vi "Database Logging.vi"() -> ()   [LabVIEW 2011]
doc: "This example inserts data into a table named logging in the LabVIEW.mdb database. The data is generated and inserted into the database once per second until you press the Stop button. You can use either of the Playback examples to read the data back into LabVIEW.\n\nThe diagram is easy to use because you only need three Database Tools subVIs - DB Tools Open Connection, DB Tools Insert Data, and DB Tools Close Connection. To insert the data, you do not need to use SQL commands or worry about defining or converting data types. You bundle all the data into a cluster and wire that cluster to the DB Tools Insert Data VI."
uses:
  <vilib>/addons/database/Connection.llb/DB Tools Open Connec (Path).vi
  <vilib>/addons/database/NI_Database_API.lvlib
panel:
  out "Number of Records":i32
  in  "stop":bool
  out "min temperature value":dbl format="%.2f"
  out "max temperature value":dbl format="%.2f"
  out "min pressure value":dbl format="%.2f"
  out "max pressure value":dbl format="%.2f"
  out "Core Temperature":dbl[](graph)
  out "Core Pressure":dbl[](graph)
  out "Core Measuments":dbl[][](graph)
  # "INSTRUCTIONS:\n\nRun the VI to insert data \ninto a table called logging \nin the example database - \nLabVIEW.mdb.  \nYou can then use the \nPlayback VIs to read the \ndata back into LabVIEW."
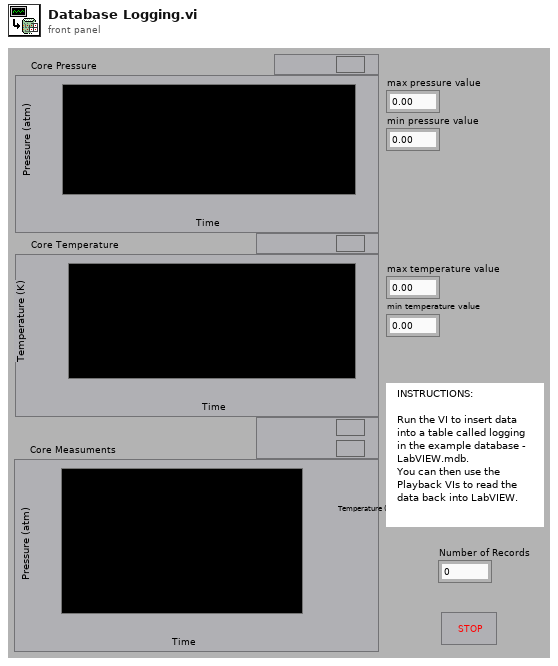
[diagram p1: front panel]
types:
  T1 = typedef "NI_Database_API.lvlib/Conn ObjectReference.ctl" = refnum<k1>
  T2 = cluster{i32, "core pressure":dbl[], dbl, dbl, "core temperature":dbl[], dbl, dbl}
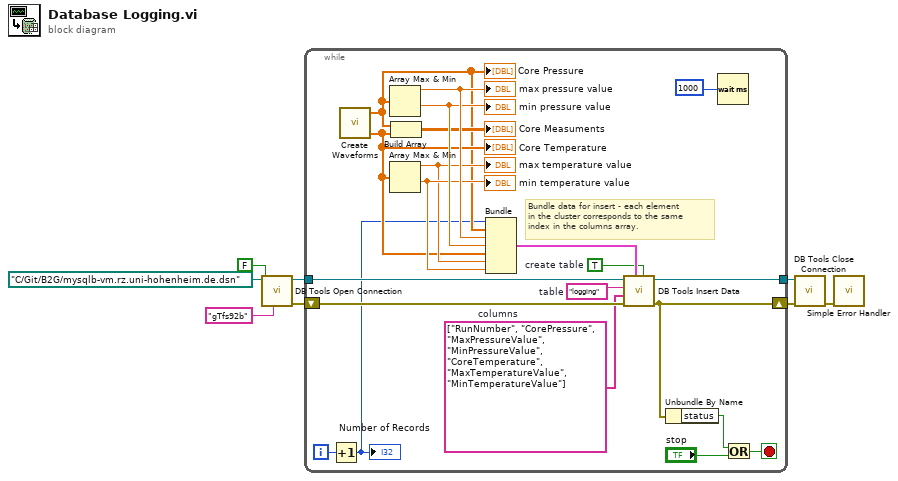
[diagram p0: block diagram]
diagram:
  n1 = call-poly <vilib>:"DB Tools Open Connection.vi"("password"="gTfs92b", "prompt? (F)"=FALSE, "connection information"=path "C:/Git/B2G/mysqlb-vm.rz.uni-hohenheim.de.dsn") -> ("error out"=w7:errorcluster, "connection reference"=w8:T1)  [unwired: 5 in]
  n2 = while {
    tunnel: w8 -> [w22]
    tunnel: [w23] -> w6
    shift-right: [w17] -> w5
    shift-left: w7 -> [w21]
    i -> [w24]
    stop <- w14 stop-if-true
    w9 = string[] ["RunNumber", "CorePressure", "MaxPressureValue", "MinPressureValue", "CoreTemperature", "MaxTemperatureValue", "MinTemperatureValue"]  # columns
    w20 = "logging"  # table
    w18 = TRUE  # create table
    # "Bundle data for insert - each element \nin the cluster corresponds to the same \nindex in the columns array."
    n3 = Increment(x=w24) -> (x+1=w10:i32)
    "Number of Records" <- w10
    n4 = call "Create Waveforms.vi"() -> ("core pressure"=w11:dbl[], "core temperature"=w12:dbl[])  [unwired: 3 in]
    "Core Pressure" <- w11
    "Core Temperature" <- w12
    n5 = Array Max & Min(array=w11) -> (max value=w29:dbl, min value=w28:dbl)  [unwired: 2 out]
    "max pressure value" <- w29
    "min pressure value" <- w28
    n6 = Array Max & Min(array=w12) -> (max value=w25:dbl, min value=w27:dbl)  [unwired: 2 out]
    "max temperature value" <- w25
    "min temperature value" <- w27
    n7 = Build Array(w11, w12) -> (→"Core Measuments":dbl[][])
    n8 = Bundle(w10, "core pressure"=w11, w29, w28, "core temperature"=w12, w25, w27) -> (w19:T2)  [unwired: 1 in]
    n9 = call <vilib>:"DB Tools Insert Data.vi"("create table? (F)"=w18, "data"=w19, "error in (no error)"=w21, "columns"=w9, "table"=w20, "connection reference"=w22) -> ("error out"=w17:errorcluster, "connection reference out"=w23:T1)  [unwired: 4 in]
    n10 = Unbundle By Name(w17) -> ("status"=w16:bool)
    n11 = Wait (ms)(milliseconds to wait=u32 1000) -> ()  [unwired: 1 out]
    n12 = Or(x=w16, y="stop") -> (x .or. y?=w14:bool)
  }
  n13 = call <vilib>:"DB Tools Close Connection.vi"("error in (no error)"=w5, "connection reference"=w6) -> ("error out"=w4:errorcluster)  [unwired: 5 in]
  n14 = call <vilib>:"Simple Error Handler.vi"("error in (no error)"=w4) -> ()  [unwired: 4 in, 5 out]
